vi "Request UI.vi"(8 "error in (no error)":errorcluster, 10 "Wait Reply":bool=TRUE, 11 "Data":cluster{"Action":string, "Data":variant}) -> (0 "error out":errorcluster, 3 "DataOut":cluster{"Action":string, "Data":variant})   [LabVIEW 2019]
uses:
  LLB/Commonly VI.lvlib
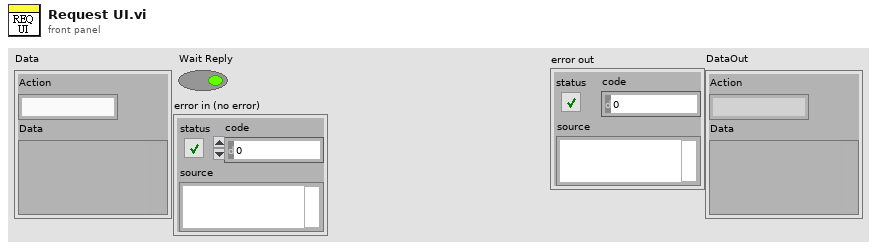
[diagram p1: front panel]
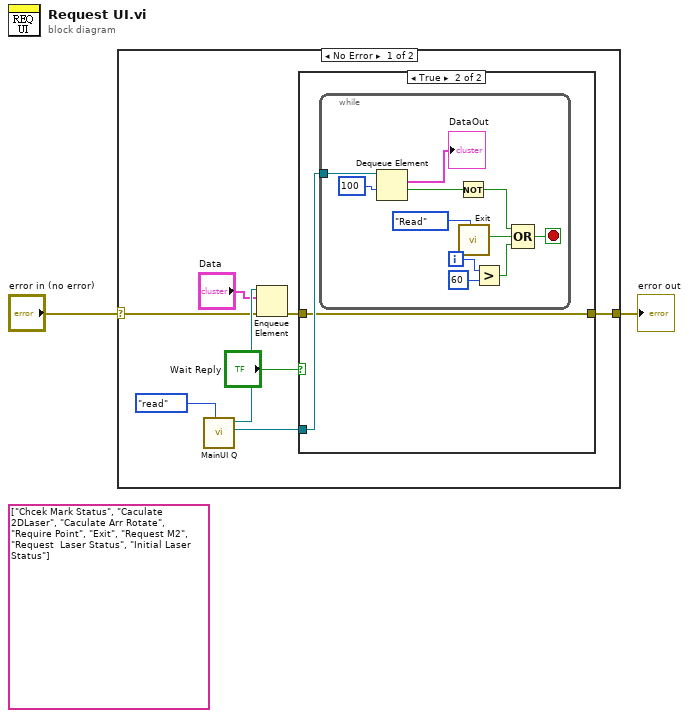
[diagram p0: block diagram]
diagram:
  (unwired) string[] ["Chcek Mark Status", "Caculate 2DLaser", "Caculate Arr Rotate", "Require Point", "Exit", "Request M2", "Request  Laser Status", "Initial Laser Status"]
  n1 = case shown="No Error" "error in (no error)" {
    selector: "error in (no error)" -> [w5 w25]
    tunnel: [w3 w25] -> w2
    frame No Error {
      n2 = call "MainUI Q.vi"("Enum"=enum16{"Initial", "read", "release"}."read") -> ("UI Response Out"=w7:refnum<queue>, "UI Receive Out"=w9:refnum<queue>)  [unwired: 9 in]
      n3 = Enqueue Element(queue=w9, element="Data", error in (no error)=w5) -> (error out=w4:errorcluster)  [unwired: 1 in, 2 out]
      n4 = case shown="True" "Wait Reply" {
        tunnel: w7 -> [_ w13]
        tunnel: w4 -> [w11 w12]
        tunnel: [w11 w12] -> w3
        frame False {
        }
        frame True {
          n5 = while {
            tunnel: w13 -> [w24]
            i -> [w16]
            stop <- w20 stop-if-true
            n6 = Dequeue Element(queue=w24, timeout in ms (-1)=100) -> (element=→"DataOut":cluster{"Action":string, "Data":variant}, timed out?=w23:bool)  [unwired: 1 in, 2 out]
            n7 = Not(x=w23) -> (.not. x?=w19:bool)
            n8 = call "Exit.vi"("Enum"=enum16{"Initial", "Read", "Write"}."Read") -> ("ExitOut"=w18:bool)  [unwired: 10 in]
            n9 = Greater?(x=w16, y=60) -> (0:w14:bool)
            n10 = Compound Arithmetic op=OR(w19, w18, w14) -> (w20:bool)
          }
        }
      }
    }
    frame Error {
    }
  }
  "error out" <- w2
